vi "Actor Core.vi"(8 "error in":errorcluster, 11 "TestStand Controller in":refnum<class "Controller API.lvclass">) -> (0 "error out":errorcluster, 3 "Actor out":refnum<class "Actor.lvclass">)   [LabVIEW 2017, in "Controller API.lvlib" / "Controller API.lvclass"]
doc: "(<B>Filename</B>: Actor Framework.lvlib:Actor.lvclass:Actor Core.vi)\n\nReceives messages to the actor, reacts to them, and initiates any error handling that may shut the actor down.\n\nDescendant classes may override this VI to append parallel tasks for the actor to complete while it handles messages. Overrides use the Call Parent Method node."
uses:
  Controller API.lvclass
  C:/Program Files (x86)/National Instruments/LabVIEW 2017/vi.lib/ActorFramework/Actor/Actor.lvclass
  <vilib>/ActorFramework/Actor/Actor.lvclass
  Controller API.lvclass/Controller API.ctl
  <vilib>/ActorFramework/Actor/Actor.lvclass/Actor.ctl
  <vilib>/ActorFramework/Message Enqueuer/Message Enqueuer.lvclass/Message Enqueuer.ctl
  <vilib>/ActorFramework/Message Enqueuer/Init from Existing Queue.vi
  <vilib>/ActorFramework/Message Enqueuer/Enqueue.vi
  <vilib>/ActorFramework/Stop Msg/Stop Msg.lvclass
  C:/Program Files (x86)/National Instruments/LabVIEW 2017/vi.lib/ActorFramework/Message/Message.lvclass
  <vilib>/ActorFramework/Message Priority Queue/Priority Enqueue.vi
  <vilib>/ActorFramework/Message Enqueuer/Message Enqueuer.lvclass
  <userlib>/Common Components/Controller/Controller.lvclass
panel:
  out "Status Window":string
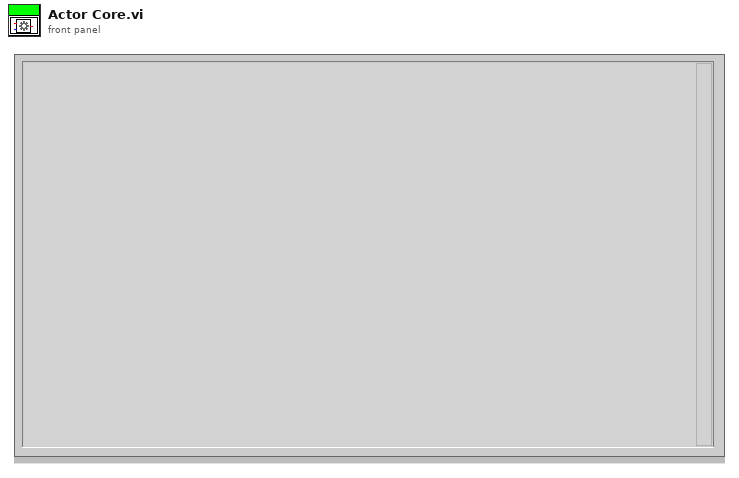
[diagram p1: front panel]
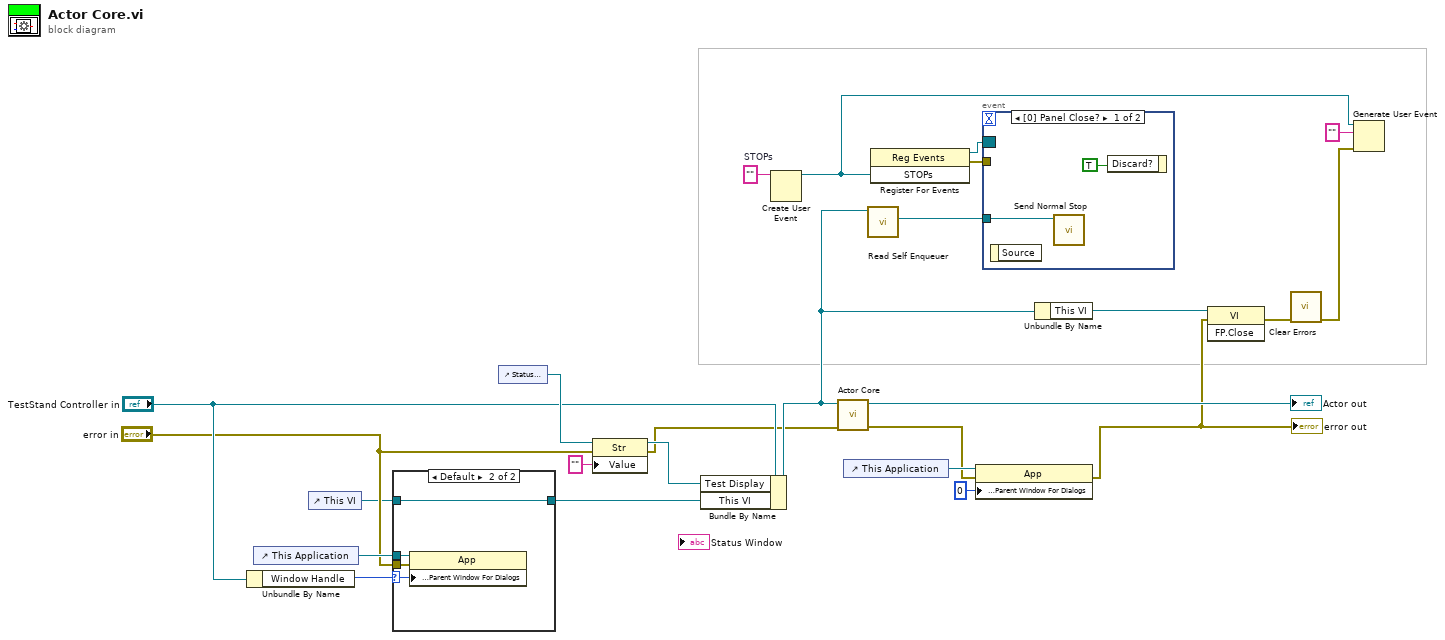
[diagram p0: block diagram]
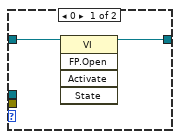
[diagram p2: hidden frame]
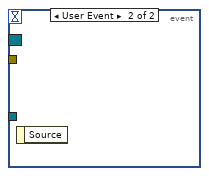
[diagram p3: hidden frame]
diagram:
  w16 = ""  # STOPs
  n1 = Unbundle By Name("TestStand Controller in") -> ("Window Handle"=w3:i32)
  n2 = control-ref of="This Application"() -> (w21:refnum<vi>)
  n3 = control-ref of="This VI"() -> (w2:refnum<vi>)
  n4 = case shown="Default" w3 {
    selector: w3 -> [_ w29]
    tunnel: w21 -> [_ w31]
    tunnel: "error in" -> [_ w30]
    tunnel: w2 -> [w27 w28]
    tunnel: [w26 w28] -> w1
    frame 0 {
      n5 = invoke class="VI" method="FP.Open"(reference=w27) -> (reference out=w26:refnum<vi>)  [unwired: 4 in, 4 out]
    }
    frame Default {
      n6 = property class="App"(reference=w31, error in=w30, "Application:Parent Window For Dialogs"=w29) -> ()  [unwired: 2 out]
    }
  }
  n7 = control-ref of="Status Window"() -> (w25:refnum<vi>)
  n8 = property class="Str"(reference=w25, error in="error in", "Value"="") -> (reference out=w22:refnum<vi>, error out=w7:errorcluster)
  n9 = Bundle By Name(cluster="TestStand Controller in", "Test Display"=w22, "This VI"=w1) -> (w19:refnum<class "Controller API.lvclass">)
  n10 = Create User Event(user event datatype=w16) -> (user event=w14:refnum<user-event>)  [unwired: 1 in, 1 out]
  n11 = call-parent "Actor Core.vi"("error in"=w7, "Controller in"=w19) -> ("error out"=w5:errorcluster, "Actor out"=→"Actor out":refnum<class "Actor.lvclass">)  [unwired: 8 in]
  n12 = control-ref of="This Application"() -> (w9:refnum<vi>)
  n13 = call <vilib>:"Read Self Enqueuer.vi"("Actor"=w19) -> ("Self Enqueuer"=w17:refnum<class "Message Enqueuer.lvclass">)  [unwired: 10 in]
  n14 = register-events(w14) -> (reference out=w15:refnum<event-registration>, error out=w12:errorcluster)  [unwired: 2 in]
  n15 = property class="App"(reference=w9, error in=w5, "Application:Parent Window For Dialogs"=0) -> (error out=w4:errorcluster)  [unwired: 1 out]
  "error out" <- w4
  n16 = event shown="[0] Panel Close?" {
    selector: w15 -> [_ _]
    dyn-events: _ -> [_ _]
    timeout: _ -> [_ _]
    tunnel: w17 -> [w33 _]
    tunnel: w12 -> [_ _]
    event Panel Close? {
      n17 = event-data() -> ()  [unwired: 1 in, 1 out]
      n18 = call <vilib>:"Send Normal Stop.vi"("Message Enqueuer"=w33) -> ()  [unwired: 10 in, 1 out]
      n19 = event-data("Discard?"=TRUE) -> ()  [unwired: 1 in, 1 out]
    }
    event User Event {
      n20 = event-data() -> ()  [unwired: 1 in, 1 out]
    }
  }
  n21 = Unbundle By Name(w19) -> ("This VI"=w18:refnum<vi>)
  n22 = invoke class="VI" method="FP.Close"(reference=w18, error in=w4) -> (error out=w11:errorcluster)  [unwired: 1 in, 2 out]
  n23 = call <vilib>:"Clear Errors.vi"("error in (no error)"=w11) -> ("error out"=w10:errorcluster)  [unwired: 5 in, 1 out]
  n24 = Generate User Event(user event=w14, event data cluster="" ("event data"), error in=w10) -> ()  [unwired: 1 in, 2 out]
